vi "sinus.vi"(8 "error in (no error)":errorcluster, 11 "dx":dbl) -> (0 "error out":errorcluster, 3 "sin(x)":dbl)   [LabVIEW 2020]
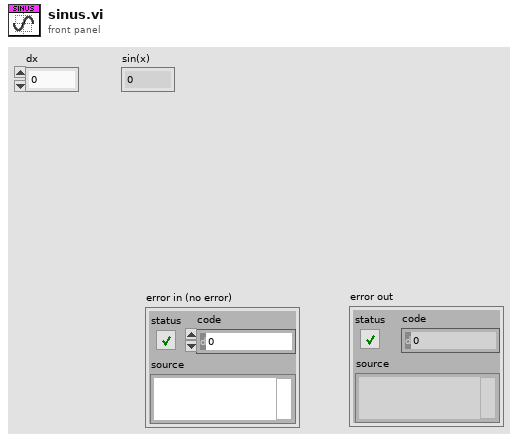
[diagram p1: front panel]
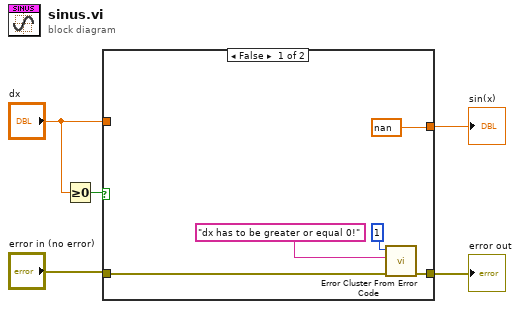
[diagram p0: block diagram]
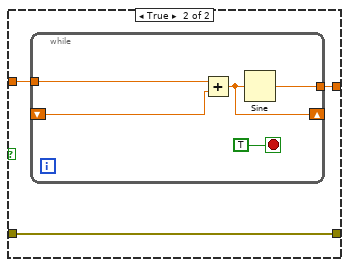
[diagram p2: hidden frame]
diagram:
  n1 = Greater Or Equal To 0?(x="dx") -> (x >= 0?=w1:bool)
  n2 = case shown="False" w1 {
    tunnel: [nan w13] -> w5
    tunnel: "dx" -> [_ w12]
    tunnel: "error in (no error)" -> [w7 w11]
    tunnel: [w6 w11] -> w2
    frame False {
      n3 = call <vilib>:"Error Cluster From Error Code.vi"("error in (no error)"=w7, "error message (\"\")"="dx has to be greater or equal 0!" ("error message (\"\")"), "error code (0)"=1) -> ("error out"=w6:errorcluster)  [unwired: 6 in]
    }
    frame True {
      n4 = while {
        shift-right: [w16] -> _
        shift-left: _ -> [w15]
        tunnel: w12 -> [w17]
        tunnel: [w14] -> w13
        stop <- TRUE stop-if-true
        n5 = Add(x=w17, y=w15) -> (x+y=w16:dbl)
        n6 = Sine(x=w16) -> (sin(x)=w14:dbl)
      }
    }
  }
  "sin(x)" <- w5
  "error out" <- w2
